vi "Setup.vi"(8 "Error In":errorcluster, 9 "Password":string, 10 "Username":string, 11 "Address":string) -> (0 "Error Out":errorcluster, 2 "Temporary File":string, 3 "SFTP":refnum<class "SFTP.lvclass">)   [LabVIEW 2018, in "Tests.lvlib" / "SFTP File.lvlib"]
uses:
  SFTP File.lvlib
  src/Toolkit/API/SFTP/SFTP.lvclass
  src/Toolkit/API/Session/Support/Password Authentication.vi
  src/Toolkit/API/SSH/SSH.lvclass
  src/Toolkit/API/Session/Session.lvclass
  Tests.lvlib
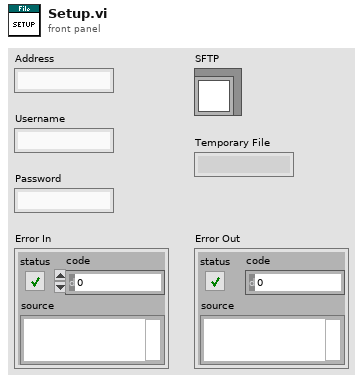
[diagram p1: front panel]
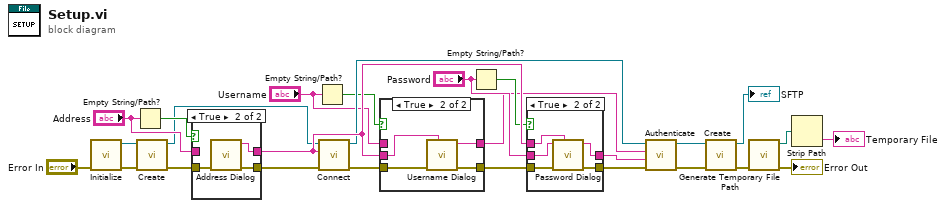
[diagram p0: block diagram]
diagram:
  n1 = call "Initialize.vi"("Error In"="Error In") -> ("Error Out"=w5:errorcluster, "SSH"=w6:refnum<class "SSH.lvclass">)  [unwired: 9 in]
  n2 = Empty String/Path?(string/path="Address") -> (empty?=w9:bool)
  n3 = call "Create.vi"("Error In"=w5, "SSH"=w6) -> ("Error Out"=w11:errorcluster, "Sesssion"=w8:refnum<class "Session.lvclass">)  [unwired: 8 in]
  n4 = case shown="True" w9 {
    tunnel: w11 -> [w27 w31]
    tunnel: [w27 w30] -> w12
    tunnel: [w28 w29] -> w26
    tunnel: "Address" -> [w28 _]
    frame False {
    }
    frame True {
      n5 = call "Address Dialog.vi"("Error In"=w31) -> ("Error Out"=w30:errorcluster, "Address Out"=w29:string)  [unwired: 9 in]
    }
  }
  n6 = Empty String/Path?(string/path="Username") -> (empty?=w19:bool)
  n7 = call "Connect.vi"("Error In"=w12, "Address"=w26, "Session In"=w8) -> ("Error Out"=w22:errorcluster, "Sesssion Out"=w25:refnum<class "Session.lvclass">)  [unwired: 7 in]
  n8 = case shown="True" w19 {
    tunnel: w22 -> [w33 w37]
    tunnel: [w32 w36] -> w17
    tunnel: [w33 w35] -> w14
    tunnel: "Username" -> [w32 _]
    tunnel: w26 -> [_ w34]
    frame False {
    }
    frame True {
      n9 = call "Username Dialog.vi"("Address"=w34, "Error In"=w37) -> ("Error Out"=w35:errorcluster, "Username Out"=w36:string)  [unwired: 8 in]
    }
  }
  n10 = Empty String/Path?(string/path="Password") -> (empty?=w21:bool)
  n11 = case shown="True" w21 {
    tunnel: "Password" -> [w39 w44]
    tunnel: w14 -> [w38 w43]
    tunnel: [w38 w42] -> w15
    tunnel: [w39 w41] -> w16
    tunnel: w26 -> [_ w40]
    frame False {
    }
    frame True {
      n12 = call "Password Dialog.vi"("Address"=w40, "Error In"=w43, "Password In"=w44) -> ("Error Out"=w42:errorcluster, "Password Out"=w41:string)  [unwired: 7 in]
    }
  }
  n13 = call-poly "Authenticate.vi"("Error In"=w15, "Password"=w16, "Username"=w17, "Session In"=w25) -> ("Error Out"=w23:errorcluster, "Sesssion Out"=w24:refnum<class "Session.lvclass">)  [unwired: 6 in]
  n14 = call "Create.vi"("Error In"=w23, "Session"=w24) -> ("Error Out"=w3:errorcluster, "SFTP"=→"SFTP":refnum<class "SFTP.lvclass">)  [unwired: 8 in]
  n15 = call <vilib>:"Generate Temporary File Path.vi"("error in (no error)"=w3) -> ("error out"=→"Error Out":errorcluster, "Unique Temporary File Path"=w4:path)  [unwired: 9 in]
  n16 = Strip Path(path=w4) -> (name=→"Temporary File":string)  [unwired: 1 out]
